vi "Key Information From Index.vi"(7 "Section Name":string="session", 8 "error in (no error)":errorcluster, 9 "Start":i32, 10 "Key Name":string="b", 11 "Config in":refnum<class "LabVIEW-Config.lvclass">) -> (0 "error out":errorcluster, 2 "Key Information":T1, 3 "Config out":refnum<class "LabVIEW-Config.lvclass">)   [LabVIEW 2017, in "LabVIEW-Config.lvlib" / "LabVIEW-Config.lvclass"]
uses:
  LabVIEW-Config.lvclass
  KeyInfo.ctl
  LabVIEW-Config.lvclass/LabVIEW-Config.ctl
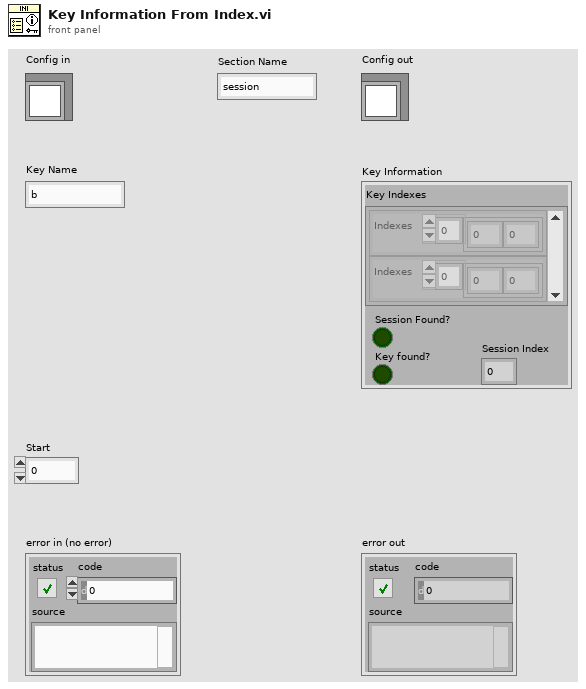
[diagram p1: front panel]
types:
  T1 = typedef "LabVIEW-Config.lvlib/LabVIEW-Config.lvclass/KeyInfo.ctl" = cluster{"Key Indexes":cluster{"Indexes":i32[]}[], "Session Found?":bool, "Key found?":bool, "Session Index":i32}
  T2 = typedef "LabVIEW-Config.lvlib/LabVIEW-Config.lvclass/LineToken.ctl" = enum8{"comment", "section", "key", "more"}
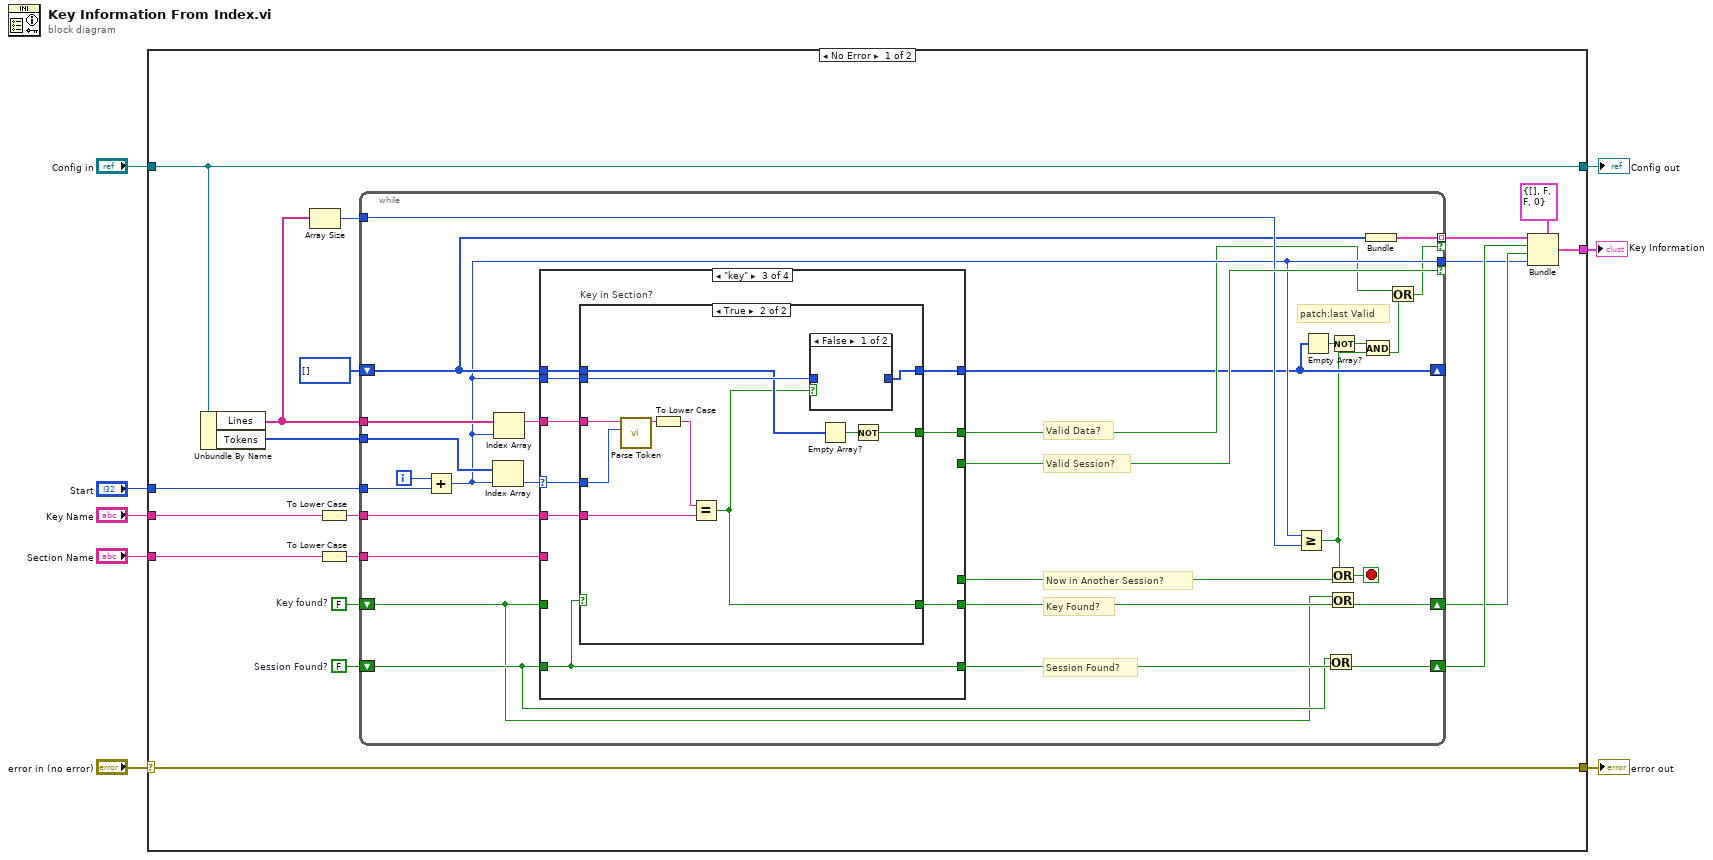
[diagram p0: block diagram]
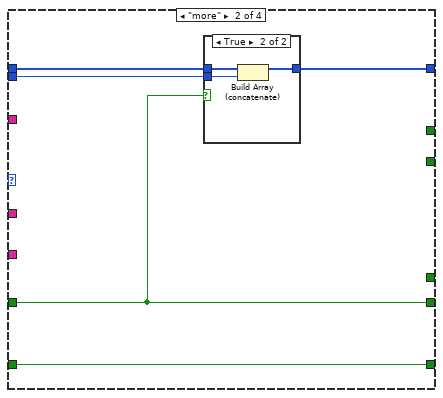
[diagram p3: hidden frame]
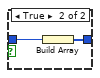
[diagram p6: hidden frame]
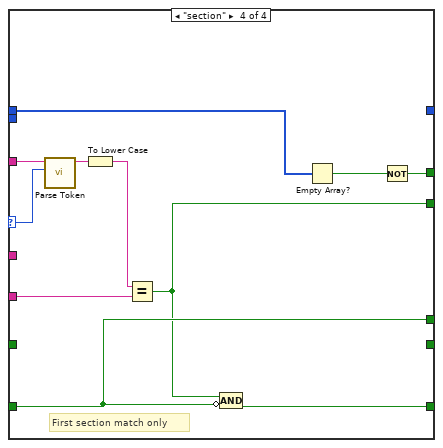
[diagram p7: hidden frame]
diagram:
  n1 = case shown="No Error" "error in (no error)" {
    selector: "error in (no error)" -> [w26 w103]
    tunnel: "Config in" -> [w14 w102]
    tunnel: [w26 w103] -> w7
    tunnel: [w14 w102] -> w5
    tunnel: "Section Name" -> [w15 _]
    tunnel: "Key Name" -> [w16 _]
    tunnel: [w20 _] -> w2
    tunnel: "Start" -> [w13 _]
    frame No Error {
      w23 = FALSE  # Key found?
      w24 = FALSE  # Session Found?
      n2 = Unbundle By Name(w14) -> ("Lines"=w11:string[], "Tokens"=w27:T2[])
      n3 = Array Size(array=w11) -> (size(s)=w10:i32)
      n4 = To Lower Case(string=w16) -> (all lower case string=w22:string)
      n5 = To Lower Case(string=w15) -> (all lower case string=w25:string)
      n6 = while {
        tunnel: w27 -> [w55]
        tunnel: w11 -> [w54]
        tunnel: w25 -> [w53]
        shift-right: [w49] -> w19
        shift-left: w24 -> [w48]
        shift-right: [w47] -> w18
        shift-left: w23 -> [w46]
        tunnel: w22 -> [w51]
        tunnel: [w38] -> w21 mode=indexing if=w33
        tunnel: w13 -> [w42]
        tunnel: [w35] -> w12 if=w41
        tunnel: w10 -> [w39]
        shift-right: [w29] -> _
        shift-left: i32[] [] ("x+y") -> [w36]
        i -> [w43]
        stop <- w40 stop-if-true
        # "patch:last Valid"
        # "Valid Session?"
        # "Valid Data?"
        # "Session Found?"
        # "Key Found?"
        # "Now in Another Session?"
        n7 = Add(x=w43, y=w42) -> (x+y=w35:i32)
        n8 = Index Array(array=w55, index=w35) -> (element=w44:T2)
        n9 = Index Array(array=w54, index=w35) -> (element=w45:string)
        n10 = case shown="\"key\"" w44 {
          selector: w44 -> [_ _ w73 w97]
          tunnel: w45 -> [_ _ w76 w98]
          tunnel: w53 -> [_ _ _ w101]
          tunnel: [w58 w63 w75 w99] -> w52
          tunnel: w48 -> [w58 w63 w75 w95]
          tunnel: w51 -> [_ _ w74 _]
          tunnel: [w57 w60 w69 _] -> w50
          tunnel: w46 -> [w57 w60 _ _]
          tunnel: [_ _ _ w95] -> w37
          tunnel: [_ _ _ w94] -> w41
          tunnel: w36 -> [w56 w62 w71 w92]
          tunnel: [w56 w61 w72 _] -> w29
          tunnel: [_ _ w70 w91] -> w34
          tunnel: w35 -> [_ w59 w68 _]
          frame "comment" {
          }
          frame "more" {
            n11 = case shown="True" w60 {
              tunnel: w62 -> [w64 w67]
              tunnel: [w64 w66] -> w61
              tunnel: w59 -> [_ w65]
              frame False {
              }
              frame True {
                n12 = Build Array (concatenate)(w67, w65) -> (w66:i32[])
              }
            }
          }
          frame "key" {
            n13 = case "Key in Section?" shown="True" w75 {
              tunnel: w76 -> [_ w86]
              tunnel: w74 -> [_ w88]
              tunnel: [_ w78] -> w69
              tunnel: w73 -> [_ w85]
              tunnel: [w77 w83] -> w72
              tunnel: w71 -> [w77 w79]
              tunnel: [_ w80] -> w70
              tunnel: w68 -> [_ w82]
              frame False {
              }
              frame True {
                n14 = call "Parse Token.vi"("Token"=w85, "Line"=w86) -> ("Name"=w84:string)  [unwired: 8 in, 1 out]
                n15 = To Lower Case(string=w84) -> (all lower case string=w87:string)
                n16 = Equal?(x=w87, y=w88) -> (x = y?=w78:bool)
                n17 = case shown="False" w78 {
                  tunnel: [_ w90] -> w83
                  tunnel: w82 -> [_ w89]
                  frame False {
                  }
                  frame True {
                    n18 = Build Array(w89) -> (w90:i32[])
                  }
                }
                n19 = Empty Array?(array=w79) -> (empty?=w81:bool)
                n20 = Not(x=w81) -> (.not. x?=w80:bool)
              }
            }
          }
          frame "section" {
            # "First section match only"
            n21 = call "Parse Token.vi"("Token"=w97, "Line"=w98) -> ("Name"=w96:string)  [unwired: 8 in, 1 out]
            n22 = To Lower Case(string=w96) -> (all lower case string=w100:string)
            n23 = Equal?(x=w100, y=w101) -> (x = y?=w94:bool)
            n24 = Compound Arithmetic op=AND(w94, invert w95) -> (w99:bool)
            n25 = Empty Array?(array=w92) -> (empty?=w93:bool)
            n26 = Not(x=w93) -> (.not. x?=w91:bool)
          }
        }
        n27 = Greater Or Equal?(x=w35, y=w39) -> (x >= y?=w28:bool)
        n28 = Empty Array?(array=w29) -> (empty?=w32:bool)
        n29 = Or(x=w48, y=w52) -> (x .or. y?=w49:bool)
        n30 = Or(x=w28, y=w37) -> (x .or. y?=w40:bool)
        n31 = Or(x=w46, y=w50) -> (x .or. y?=w47:bool)
        n32 = Not(x=w32) -> (.not. x?=w30:bool)
        n33 = And(x=w30, y=w28) -> (x .and. y?=w31:bool)
        n34 = Bundle("x+y"=w36) -> (w38:cluster{"x+y":i32[]})  [unwired: 1 in]
        n35 = Or(x=w34, y=w31) -> (x .or. y?=w33:bool)
      }
      n36 = Bundle(cluster=T1 {"Key Indexes"=[], "Session Found?"=FALSE, "Key found?"=FALSE, "Session Index"=0}, "Key Indexes"=w21, "Session Found?"=w19, "Key found?"=w18, "Session Index"=w12) -> (w20:T1)
    }
    frame Error {
    }
  }
  "error out" <- w7
  "Config out" <- w5
  "Key Information" <- w2
